vi "Analogue_overflow_checker.vi"(2 "I16 data":i16[][](array[numeric])) -> (0 "Over/Under string":string)   [LabVIEW 2010]
uses:
  Globals/Meas_global.vi
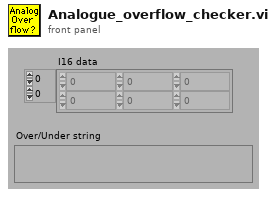
[diagram p1: front panel]
types:
  T1 = typedef "Board_Types.ctl" = enum16{"Simulate", "NB-MIO-16H", "PCI-MIO-16E", "6000E Series", "USB-92xx", "ADC488", "Lab-NB", "NB-DIO-24", "NI-DAQmx", "Local ADAM", "Server Channels"}
  T2 = typedef "Ch_and_Spans.ctl" = cluster{"high limit (10V)":sgl, "low limit (-10V)":sgl, "Ch No":i16, "Var name":string, "Use Latest Calib":bool}
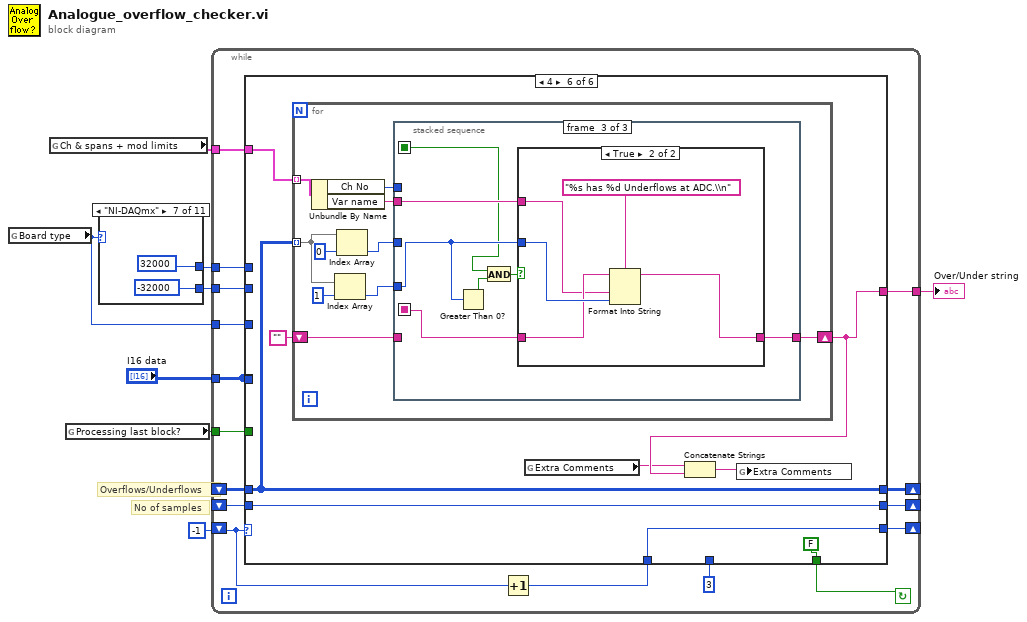
[diagram p0: block diagram]
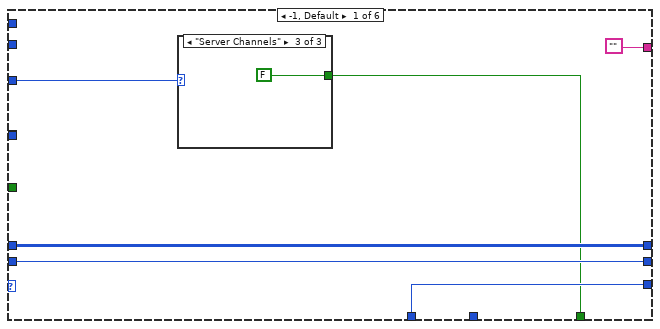
[diagram p2: hidden frame]
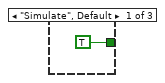
[diagram p3: hidden frame]
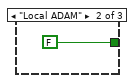
[diagram p4: hidden frame]
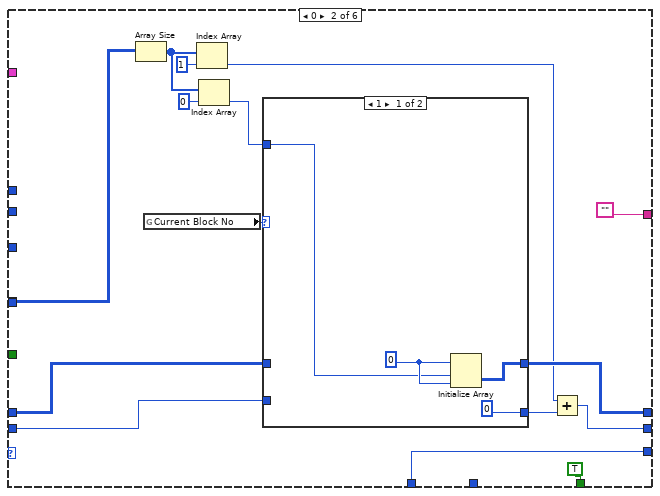
[diagram p5: hidden frame]
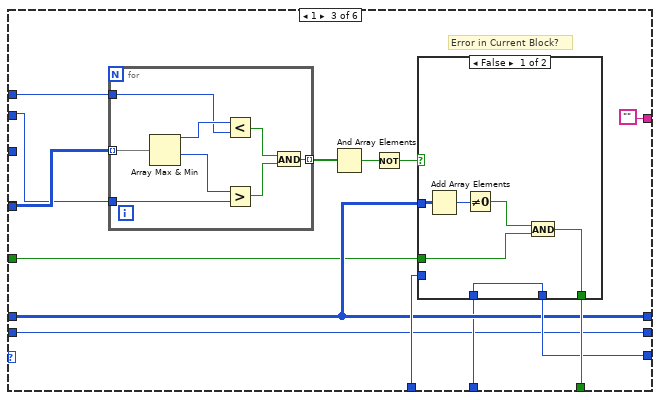
[diagram p7: hidden frame]
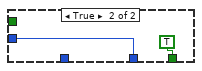
[diagram p8: hidden frame]
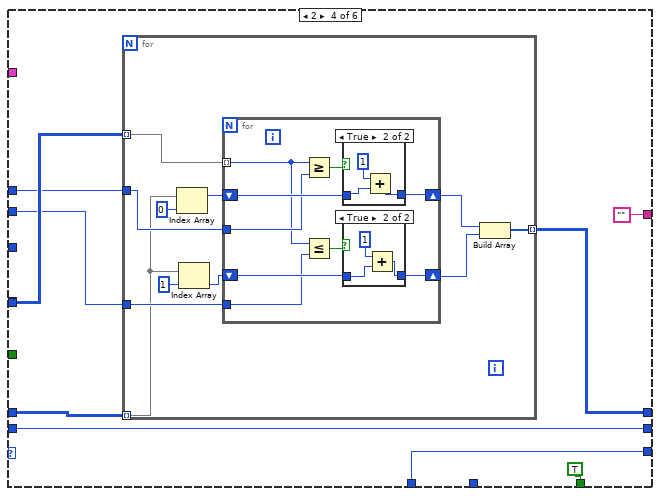
[diagram p9: hidden frame]
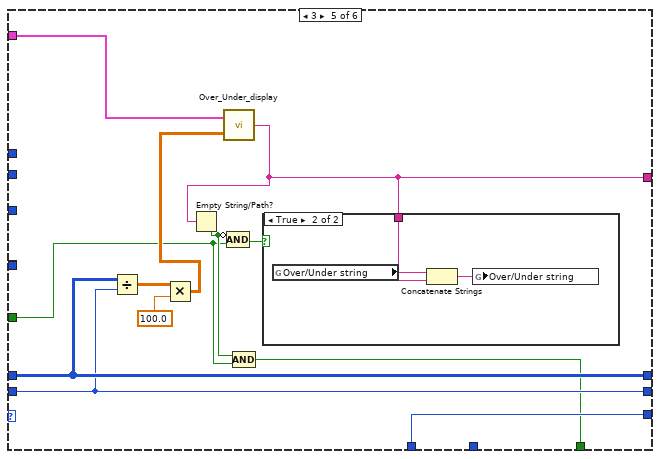
[diagram p12: hidden frame]
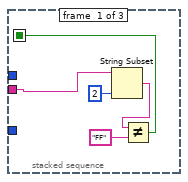
[diagram p14: hidden frame]
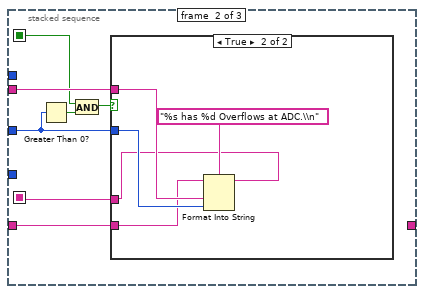
[diagram p15: hidden frame]
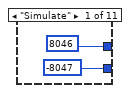
[diagram p18: hidden frame]
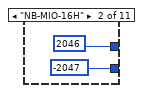
[diagram p19: hidden frame]
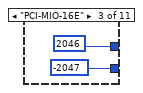
[diagram p20: hidden frame]
diagram:
  # "No of samples"
  # "Overflows/Underflows"
  n1 = global read "Meas_global.vi" "Board type"() -> (w2:T1)
  n2 = global read "Meas_global.vi" "Ch & spans + mod limits"() -> (w1:T2[])
  n3 = global read "Meas_global.vi" "Processing last block?"() -> (w4:bool)
  n4 = case shown="\"NI-DAQmx\"" w2 {
    tunnel: [i16 8046 i16 2046 i16 2046 i16 31500 i16 31500 i16 31500 i16 32000 i16 2046 i16 2046 i16 32765 i16 32765] -> w8
    tunnel: [i16 -8047 i16 -2047 i16 -2047 i16 -31500 i16 -31500 i16 -31500 i16 -32000 i16 -2047 i16 -2047 i16 -32765 i16 -32765] -> w7
    frame "Simulate" {
    }
    frame "NB-MIO-16H" {
    }
    frame "PCI-MIO-16E" {
    }
    frame "ADC488" {
    }
    frame "6000E Series" {
    }
    frame "USB-92xx" {
    }
    frame "NI-DAQmx" {
    }
    frame "Lab-NB" {
    }
    frame "NB-DIO-24" {
    }
    frame "Local ADAM" {
    }
    frame "Server Channels" {
    }
  }
  n5 = while {
    tunnel: w2 -> [w31]
    tunnel: [w32] -> w3
    tunnel: w4 -> [w34]
    shift-left: _ -> [w38]
    shift-right: [w35] -> _
    shift-left: _ -> [w37]
    shift-right: [w36] -> _
    tunnel: "I16 data" -> [w39]
    shift-left: -1 -> [w42]
    shift-right: [w40] -> _
    tunnel: w7 -> [w44]
    tunnel: w8 -> [w45]
    tunnel: w1 -> [w46]
    stop <- w43 continue-if-true
    n6 = Increment(x=w42) -> (x+1=w41:i32)
    n7 = case shown="4" w42 {
      tunnel: w46 -> [_ _ _ _ w154 w162]
      tunnel: w45 -> [_ _ w89 w113 _ _]
      tunnel: w44 -> [_ _ w88 w114 _ _]
      tunnel: w39 -> [_ w62 w90 _ _ _]
      tunnel: [w47 TRUE w85 TRUE w144 FALSE] -> w43
      tunnel: w41 -> [w49 w65 w83 w111 w155 w167]
      tunnel: [w49 w65 w84 w111 w155 w167] -> w40
      tunnel: w39 -> [_ _ _ w115 _ _]
      tunnel: w38 -> [w50 w68 w79 w107 w152 w166]
      tunnel: w37 -> [w51 w66 w82 w108 w153 w163]
      tunnel: [w51 w69 w82 w112 w153 w163] -> w36
      tunnel: [w50 w59 w79 w107 w152 w166] -> w35
      tunnel: w34 -> [_ _ w77 _ w145 _]
      tunnel: 3 -> [_ _ w81 _ _ _]
      tunnel: ["" "" "" "" w147 w160] -> w32
      tunnel: w31 -> [w48 _ _ _ _ _]
      frame -1, Default {
        n8 = case shown="\"Server Channels\"" w48 {
          tunnel: [TRUE FALSE FALSE] -> w47
          frame "Simulate", Default {
          }
          frame "Local ADAM" {
          }
          frame "Server Channels" {
          }
        }
      }
      frame 0 {
        n9 = Array Size(array=w62) -> (size(s)=w57:i32[])
        n10 = global read "Meas_global.vi" "Current Block No"() -> (w70:i32)
        n11 = Index Array(array=w57, index=1 ("Index")) -> (element=w61:i32)
        n12 = Index Array(array=w57, index=0 ("Index")) -> (element=w56:i32)
        n13 = case shown="1" w70 {
          tunnel: [w74 w76] -> w69
          tunnel: w66 -> [_ w76]
          tunnel: w68 -> [_ w75]
          tunnel: [0 w75] -> w60
          tunnel: w56 -> [w71 _]
          frame 1 {
            w72 = 0
            n14 = Initialize Array(w72, w71, w72) -> (w74:i32[][])
          }
          frame 2, Default {
          }
        }
        n15 = Add(x=w61, y=w60) -> (x+y=w59:i32)
      }
      frame 1 {
        # "Error in Current Block?"
        n16 = for {
          tunnel: w90 -> [w106] mode=indexing
          tunnel: w89 -> [w104]
          tunnel: w88 -> [w102]
          tunnel: [w99] -> w87 mode=indexing
          n17 = Array Max & Min(array=w106) -> (max value=w105:i16, min value=w103:i16)  [unwired: 2 out]
          n18 = Less?(x=w105, y=w104) -> (x < y?=w100:bool)
          n19 = Greater?(x=w103, y=w102) -> (0:w101:bool)
          n20 = And(x=w100, y=w101) -> (x .and. y?=w99:bool)
        }
        n21 = And Array Elements(Boolean array=w87) -> (logical AND=w86:bool)
        n22 = Not(x=w86) -> (.not. x?=w78:bool)
        n23 = case shown="False" w78 {
          tunnel: [w92 TRUE] -> w85
          tunnel: [w91 w97] -> w84
          tunnel: w83 -> [_ w97]
          tunnel: w82 -> [w96 _]
          tunnel: w81 -> [w91 _]
          tunnel: w77 -> [w93 _]
          frame False {
            n24 = Add Array Elements(numeric array=w96) -> (sum=w95:i32)
            n25 = Not Equal To 0?(x=w95) -> (x != 0?=w94:bool)
            n26 = And(x=w94, y=w93) -> (x .and. y?=w92:bool)
          }
          frame True {
          }
        }
      }
      frame 2 {
        n27 = for {
          tunnel: w115 -> [w124] mode=indexing
          tunnel: w114 -> [w126]
          tunnel: w113 -> [w125]
          tunnel: [w122] -> w112 mode=indexing
          tunnel: w108 -> [w118] mode=indexing
          n28 = Index Array(array=w118, index=0 ("Index")) -> (element=w116:i32)
          n29 = Index Array(array=w118, index=1 ("Index")) -> (element=w117:i32)
          n30 = for {
            shift-right: [w130] -> w121
            shift-left: w117 -> [w131]
            shift-right: [w133] -> w123
            shift-left: w116 -> [w134]
            tunnel: w124 -> [w127] mode=indexing
            tunnel: w126 -> [w129]
            tunnel: w125 -> [w128]
            n31 = Greater Or Equal?(x=w127, y=w128) -> (x >= y?=w135:bool)
            n32 = Less Or Equal?(x=w127, y=w129) -> (x <= y?=w132:bool)
            n33 = case shown="True" w135 {
              tunnel: [w140 w142] -> w133
              tunnel: w134 -> [w140 w143]
              frame False {
              }
              frame True {
                n34 = Add(x=1, y=w143) -> (x+y=w142:i32)
              }
            }
            n35 = case shown="True" w132 {
              tunnel: w131 -> [w136 w138]
              tunnel: [w136 w137] -> w130
              frame False {
              }
              frame True {
                n36 = Add(x=1, y=w138) -> (x+y=w137:i32)
              }
            }
          }
          n37 = Build Array(w123, w121) -> (w122:i32[])
        }
      }
      frame 3 {
        n38 = Divide(x=w153, y=w152) -> (x/y=w151:dbl[][])
        n39 = Multiply(x=w151, y=100.0) -> (x*y=w149:dbl[][])
        n40 = call "Over_Under_display.vi"("Overflow array"=w149, "Ch & spans"=w154) -> ("Over/Under string"=w147:string)
        n41 = Empty String/Path?(string/path=w147) -> (empty?=w146:bool)
        n42 = Compound Arithmetic op=AND(invert w146, w145) -> (w148:bool)
        n43 = Compound Arithmetic op=AND(w146, w145) -> (w144:bool)
        n44 = case shown="True" w148 {
          tunnel: w147 -> [_ w156]
          frame False {
          }
          frame True {
            n45 = global read "Meas_global.vi" "Over/Under string"() -> (w158:string)
            n46 = Concatenate Strings(w158, w156) -> (w157:string)
            n47 = global write "Meas_global.vi" "Over/Under string"(w157) -> ()
          }
        }
      }
      frame 4 {
        n48 = for {
          tunnel: w162 -> [w177] mode=indexing
          tunnel: w163 -> [w176] mode=indexing
          shift-right: [w168] -> w160
          shift-left: "" -> [w169]
          n49 = Unbundle By Name(w177) -> ("Ch No"=w175:i16, "Var name"=w174:string)
          n50 = Index Array(array=w176, index=1) -> (element=w170:i32)
          n51 = Index Array(array=w176, index=0) -> (element=w171:i32)
          n52 = stacked-sequence {
            seq-local: [_ w187 _] -> [_ _ w202]
            seq-local: [w178 _ _] -> [_ w184 w196]
            tunnel: w170 -> [_ _ w200]
            tunnel: w171 -> [_ w186 _]
            tunnel: w174 -> [w179 w189 w199]
            tunnel: w175 -> [_ _ _]
            tunnel: w169 -> [_ w188 _]
            tunnel: [_ _ w201] -> w168
            frame #0 {
              n53 = String Subset(string=w179, length (rest)=2 ("length (rest)")) -> (substring=w181:string)  [unwired: 1 out]
              n54 = Not Equal?(x=w181, y="FF") -> (x != y?=w178:bool)
            }
            frame #1 {
              n55 = Greater Than 0?(x=w186) -> (x > 0?=w185:bool)
              n56 = And(x=w184, y=w185) -> (x .and. y?=w183:bool)
              n57 = case shown="True" w183 {
                tunnel: w186 -> [_ w193]
                tunnel: w189 -> [_ w194]
                tunnel: w188 -> [w190 w192]
                tunnel: [w190 w191] -> w187
                frame False {
                }
                frame True {
                  n58 = Format Into String(format string="%s has %d Overflows at ADC.\\n" ("Format String"), initial string=w192, w194, w193) -> (resulting string=w191:string)  [unwired: 1 in, 1 out]
                }
              }
            }
            frame #2 {
              n59 = Greater Than 0?(x=w200) -> (x > 0?=w198:bool)
              n60 = And(x=w196, y=w198) -> (x .and. y?=w197:bool)
              n61 = case shown="True" w197 {
                tunnel: w200 -> [_ w208]
                tunnel: w199 -> [_ w204]
                tunnel: w202 -> [w203 w207]
                tunnel: [w203 w206] -> w201
                frame False {
                }
                frame True {
                  n62 = Format Into String(format string="%s has %d Underflows at ADC.\\n" ("Format String"), initial string=w207, w204, w208) -> (resulting string=w206:string)  [unwired: 1 in, 1 out]
                }
              }
            }
          }
        }
        n63 = global read "Meas_global.vi" "Extra Comments"() -> (w159:string)
        n64 = Concatenate Strings(w159, w160) -> (w164:string)
        n65 = global write "Meas_global.vi" "Extra Comments"(w164) -> ()
      }
    }
  }
  "Over/Under string" <- w3
